vi "ClearLimits.vi"(0 "Interface in":T1, 11 "error in (no error)":errorcluster) -> (4 "Interface out":T1, 15 "error out":errorcluster)   [LabVIEW 2016, in "ScaleAndLimitInterface.lvlib"]
uses:
  ScaleAndLimitInterface.lvlib
  Interface.ctl
  <instrlib>/_niInstr/Instruction Framework/v1/Host/Instruction Framework Context/niInstr Instruction Framework Context v1 Host.lvclass
  <instrlib>/_niInstr/Instruction Framework/v1/Host/Instruction Target/niInstr Instruction Target v1 Host.lvclass
  Configuration.ctl
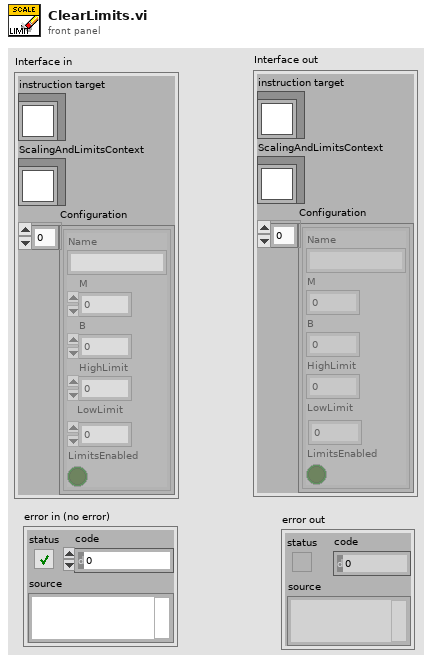
[diagram p1: front panel]
types:
  T1 = typedef "ScaleAndLimitInterface.lvlib/Interface.ctl" = cluster{"instruction target":refnum<class "niInstr Instruction Target v1 Host.lvclass">, "ScalingAndLimitsContext":refnum<class "niInstr Instruction Framework Context v1 Host.lvclass">, "Configuration":T2[]}
  T2 = typedef "ScaleAndLimitInterface.lvlib/Configuration.ctl" = cluster{"Name":string, "M":dbl, "B":i16, "HighLimit":dbl, "LowLimit":dbl, "LimitsEnabled":bool}
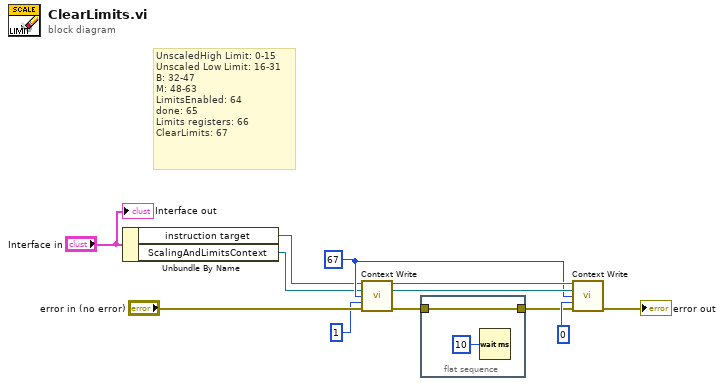
[diagram p0: block diagram]
diagram:
  w4 = u64 67 ("address")
  # "UnscaledHigh Limit: 0-15\nUnscaled Low Limit: 16-31\nB: 32-47\nM: 48-63\nLimitsEnabled: 64\ndone: 65\nLimits registers: 66\nClearLimits: 67"
  n1 = Unbundle By Name("Interface in") -> ("instruction target"=w3:refnum<class "niInstr Instruction Target v1 Host.lvclass">, "ScalingAndLimitsContext"=w2:refnum<class "niInstr Instruction Framework Context v1 Host.lvclass">)
  n2 = call <instrlib>:"Context Write.vi"("instruction target in"=w3, "context in"=w2, "address"=w4, "data"=u64 1, "error in"="error in (no error)") -> ("instruction target out"=w12:refnum<class "niInstr Instruction Target v1 Host.lvclass">, "context out"=w11:refnum<class "niInstr Instruction Framework Context v1 Host.lvclass">, "error out"=w7:errorcluster)  [unwired: 8 in]
  n3 = flat-sequence {
    tunnel: w7 -> [w14]
    tunnel: [w14] -> w6
    frame #0 {
      n4 = Wait (ms)(milliseconds to wait=u32 10) -> ()  [unwired: 1 out]
    }
  }
  n5 = call <instrlib>:"Context Write.vi"("instruction target in"=w12, "context in"=w11, "address"=w4, "data"=u64 0, "error in"=w6) -> ("error out"=→"error out":errorcluster)  [unwired: 8 in, 2 out]
  "Interface out" <- "Interface in"
